vi "Load_Traverse_file.vi"(0 "Setup filename":path) -> (2 "Fast Plotting?":bool, 3 "Setup filename Out":path, 5 "Table":T2[](array[typedef]) {"Carrier_2 Q (l/min)" format="%#.2f"; "Row Duration (mins)" format="%#.1f"; "Row No" min=0; "Trace Gas Concentration (%)" min=0.0 format="%#_4f"; "Carrier_1 Q (l/min)" format="%#.4f"; "Start X" format="%#.2f"; "Start Y" format="%#.2f"; "Start Z" format="%#.2f"; "End X" format="%#.2f"; "End Y" format="%#.2f"; "End Z" format="%#.2f"; "Tunnel Speed" format="%#.2f"; "Averaging time (mins)" min=0.0 format="%#.2f"}, 6 "Work in Tunnel Coordinates?":T1)   [LabVIEW 2020]
uses:
  Traverse_cluster.ctl
  Spacing.ctl
  Controls/Multi_run_mode.ctl
  Controls/Tunnel_Coordinates.ctl
panel:
  # "HD:Users"
  # "HD:Users"
  # "X           Y          Z"
  # "Start"
  # "End"
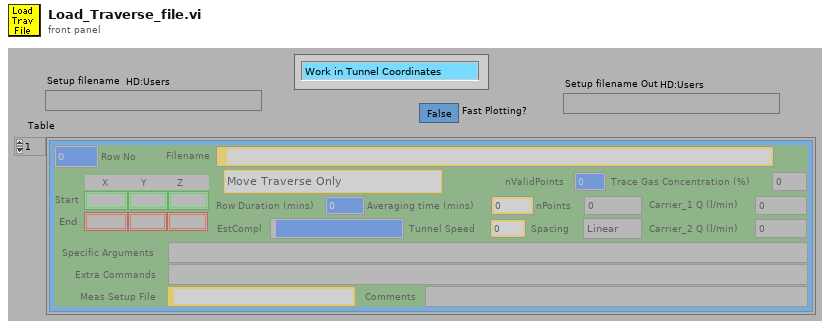
[diagram p1: front panel]
types:
  T1 = typedef "Tunnel_Coordinates.ctl" = enum16{"Work in Tunnel Coordinates", "Work in Model Coordinates"}
  T2 = typedef "Traverse_cluster.ctl" = cluster{"Start X":sgl, "Start Y":sgl, "Start Z":sgl, "End X":sgl, "End Y":sgl, "End Z":sgl, "nPoints":i32, "Spacing":T3, "Filename":path, "Tunnel Speed":dbl, "Averaging time (mins)":dbl, "Extra Commands":string, "Carrier_1 Q (l/min)":dbl, "Carrier_2 Q (l/min)":dbl, "Trace Gas Concentration (%)":dbl, "Specific Arguments":string, "Comments":string, "Row No":i32, "Row Type Selector":T4, "EstCompl":string, "Row Duration (mins)":dbl, "nValidPoints":i32, "Meas Setup File":string}
  T3 = typedef "Spacing.ctl" = enum16{"Linear", "Log", "Gauss", "Specified", "N/A"}
  T4 = typedef "Multi_run_mode.ctl" = enum16{"Move Traverse Only", "Set Tunnel Speed Only", "Set Source Only", "Set Measurement Conditions", "Single Measurement", "Vertical Profile", "Lateral Profile", "Longitudinal Profile", "Multi-Axis Profile", "Explore Volume", "Auto Calibrate", "Meas Fast FID Bkgnd", "Check Beam Power", "Scanning Valve Measurement", "Run VI Named:", "Set ADAM Ch", "Wait (minutes)", "Send Message", "Synchronize With:", "Fall Back to this Row", "Turn Off Row Repeating", "Traverse 3D Volume", "Blank Row", "Jump to Fall Back Row"}
  T5 = enum16{"All Channel Names", "Valid Channel Names"}
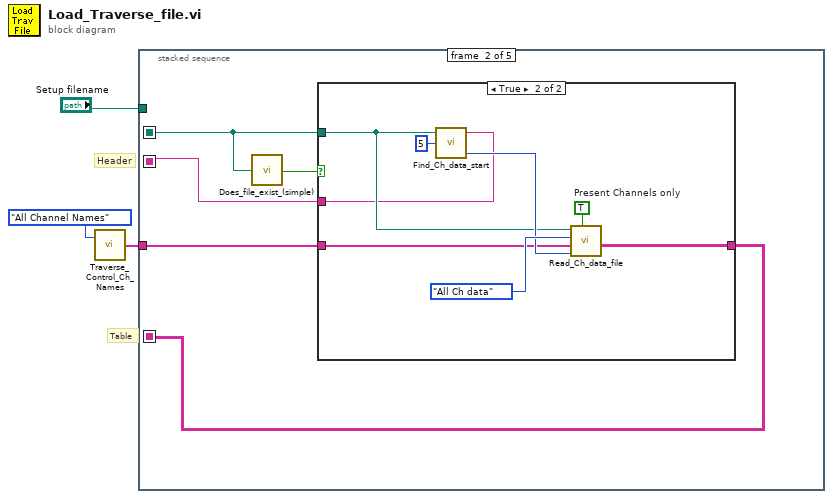
[diagram p0: block diagram]
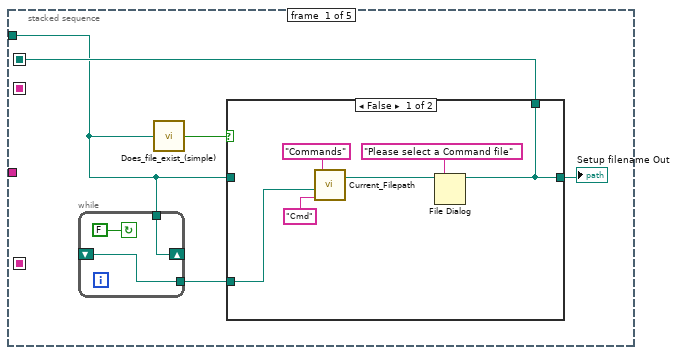
[diagram p2: hidden frame]
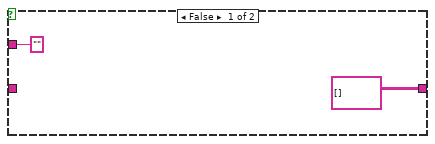
[diagram p4: hidden frame]
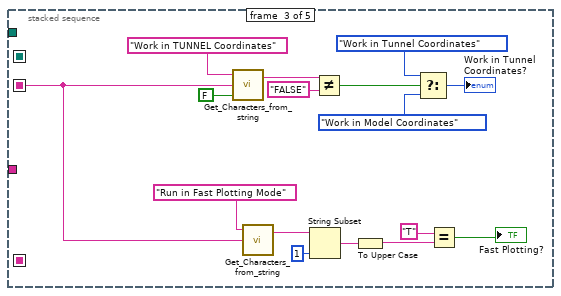
[diagram p5: hidden frame]
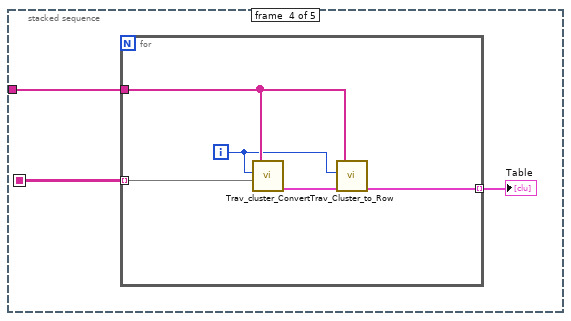
[diagram p6: hidden frame]
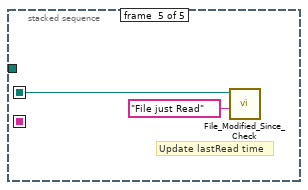
[diagram p7: hidden frame]
diagram:
  # "Header"
  # "Table"
  n1 = call "Traverse_Control_Ch_Names.vi"("Mode"=T5."All Channel Names") -> ("Channel names"=w2:string[])  [unwired: 1 in]
  n2 = stacked-sequence {
    seq-local: [_ w23 _ _ _] -> [_ _ _ w52 _]
    seq-local: [_ w22 _ _ _] -> [_ _ w35 _ _]
    seq-local: [w8 _ _ _ _] -> [_ w20 _ _ w59]
    tunnel: "Setup filename" -> [w4 _ _ _ _]
    tunnel: w2 -> [_ w19 _ w51 _]
    frame #0 {
      n3 = while {
        tunnel: [w10] -> w5
        tunnel: w4 -> [w11]
        shift-left: _ -> [w10]
        shift-right: [w11] -> _
        stop <- FALSE continue-if-true
      }
      n4 = call "Does_file_exist_(simple).vi"("Pathname"=w4) -> ("exists?"=w6:bool)
      n5 = case shown="False" w6 {
        tunnel: w4 -> [_ w18]
        tunnel: [w16 w18] -> w8
        tunnel: [w16 w18] -> w7
        tunnel: w5 -> [w14 _]
        frame False {
          n6 = call "Current_Filepath.vi"("Short_Name"="Cmd" ("Data Type"), "Filename in"=w14, "Data Type"="Commands") -> ("Directory"=w13:path)  [unwired: 1 in, 1 out]
          n7 = File Dialog(7:"Please select a Command file" ("prompt"), 11:w13) -> (3:w16:path)  [unwired: 1 in, 7 out]
        }
        frame True {
        }
      }
      "Setup filename Out" <- w7
    }
    frame #1 {
      n8 = call "Does_file_exist_(simple).vi"("Pathname"=w20) -> ("exists?"=w21:bool)
      n9 = case shown="True" w21 {
        tunnel: [string[][] [] w28] -> w23
        tunnel: ["" ("character string") w29] -> w22
        tunnel: w20 -> [_ w30]
        tunnel: w19 -> [_ w27]
        frame False {
        }
        frame True {
          w33 = TRUE  # Present Channels only
          n10 = call "Find_Ch_data_start.vi"("Approx No Of Columns"=5, "Filename"=w30) -> ("Start of read offset output"=w31:i32, "String before data"=w29:string)  [unwired: 1 in, 1 out]
          n11 = call "Read_Ch_data_file.vi"("Present Channels only"=w33, "Start of read offset (chars.: 0)"=w31, "Present Channels"=w27, "Output"=enum16{"All Ch data", "The last few rows"}."All Ch data", "Filename"=w30) -> ("Channel Values"=w28:string[][])  [unwired: 4 out]
        }
      }
    }
    frame #2 {
      n12 = call "Get_Characters_from_string.vi"("Show Dialog?"=FALSE, "Input string"=w35, "Variable name"="Work in TUNNEL Coordinates" ("Label for characters")) -> ("Value"=w48:string)  [unwired: 1 out]
      n13 = call "Get_Characters_from_string.vi"("Input string"=w35, "Variable name"="Run in Fast Plotting Mode" ("Label for characters")) -> ("Value"=w41:string)  [unwired: 1 in, 1 out]
      n14 = String Subset(string=w41, length (rest)=1 ("length")) -> (substring=w39:string)  [unwired: 1 out]
      n15 = Not Equal?(x=w48, y="FALSE") -> (x != y?=w46:bool)
      n16 = To Upper Case(1:w39) -> (0:w40:string)
      n17 = Select(t=Tunnel_Coordinates."Work in Tunnel Coordinates" ("Work in Tunnel Coordinates?"), s=w46, f=Tunnel_Coordinates."Work in Model Coordinates" ("Work in Tunnel Coordinates?")) -> (s? t:f=→"Work in Tunnel Coordinates?":T1)
      n18 = Equal?(x="T", y=w40) -> (x = y?=→"Fast Plotting?":bool)
    }
    frame #3 {
      n19 = for {
        tunnel: w52 -> [w57] mode=indexing
        tunnel: [w54] -> w50 mode=indexing
        tunnel: w51 -> [w56]
        i -> [w55]
        n20 = call "Trav_cluster_Convert.vi"("Channel Values In"=w57, "Row Number"=w55, "Channel names"=w56) -> ("Traverse line Out"=w53:T2)  [unwired: 1 in, 3 out]
        n21 = call "Trav_Cluster_to_Row.vi"("Traverse line in"=w53, "Row Number"=w55, "Channel names"=w56) -> ("Traverse line Out"=w54:T2)  [unwired: 4 out]
      }
      "Table" <- w50
    }
    frame #4 {
      # "Update lastRead time"
      n22 = call "File_Modified_Since_Check.vi"("mode"="File just Read", "File Path"=w59) -> ()  [unwired: 6 in, 2 out]
    }
  }
